vi "element_data_read.vi"(7 "container_name":string, 8 "error in (no error)":errorcluster, 10 "data_type":variant, 11 "Refnum in":T1) -> (0 "error out":errorcluster, 1 "Data Name":string, 2 "data_out":variant, 3 "Refnum out":T1)   [LabVIEW 2015, in "ini_work_Library.lvlib"]
doc: "Created by Artem Shevelev\nshevelev.pro\nartem@shevelev.pro\nLabVIEW Portal: https://labviewportal.org/memberlist.php?mode=viewprofile&u=2340"
uses:
  ini_work_Library.lvlib
  <vilib>/Utility/config.llb/Config Data RefNum.ctl
  <userlib>/_OpenG.lib/lvdata/lvdata.llb/Type Descriptor Enumeration__ogtk.ctl
  <vilib>/Utility/config.llb/Read Key (I32).vi
  <vilib>/Utility/config.llb/Read Key (Double).vi
  <vilib>/Utility/config.llb/Read Key (Boolean).vi
  <vilib>/Utility/config.llb/Read Key (String).vi
  <vilib>/Utility/config.llb/Read Key (Path).vi
  <vilib>/Utility/config.llb/NI_LVConfig.lvlib
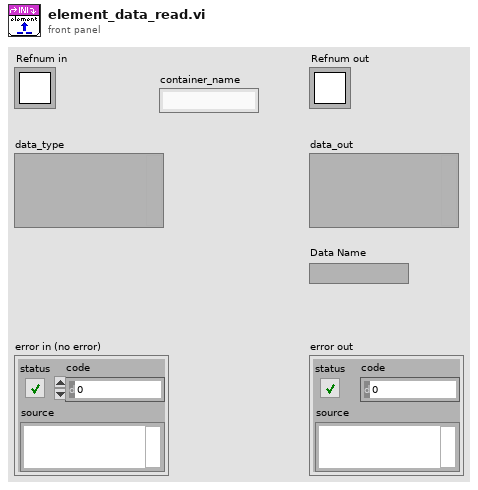
[diagram p1: front panel]
types:
  T1 = typedef "NI_LVConfig.lvlib/Config Data RefNum.ctl" = refnum<k1>
  T2 = typedef "Type Descriptor Enumeration__ogtk.ctl" = enum8{"<Null>", "I8", "I16", "I32", "I64", "U8", "U16", "U32", "U64", "SGL", "DBL", "EXT", "CSG", "CDB", "CXT", "0x0F", "0x10", "0x11", "0x12", "0x13", "0x14", "Enum U8", "Enum U16", "Enum U32", "Enum U64", "SGL PQ", "DBL PQ", "EXT PQ", "CSG PQ", "CDB PQ", "CXT PQ", "0x1F", "0x20", "Boolean", "0x22", "0x23", "0x24", "0x25", "0x26", "0x27", "0x28", "0x29", "0x2A", "0x2B", "0x2C", "0x2D", "0x2E", "0x2F", "String", "0x31", "Path", "Pict", "0x34", "0x35", "0x36", "DAQ", "0x38", "0x39", "0x3A", "0x3B", "0x3C", "0x3D", "0x3E", "0x3F", "Array", "0x41", "0x42", "0x43", "0x44", "0x45", "0x46", "0x47", "0x48", "0x49", "0x4A", "0x4B", "0x4C", "0x4D", "0x4E", "0x4F", "Cluster", "0x51", "0x52", "Variant", "Waveform", "0x55", "0x56", "0x57", "0x58", "0x59", "0x5A", "0x5B", "0x5C", "0x5D", "0x5E", "Fixed Point", "0x60", "0x61", "0x62", "0x63", "0x64", "0x65", "0x66", "0x67", "0x68", "0x69", "0x6A", "0x6B", "0x6C", "0x6D", "0x6E", "0x6F", "Refnum", "0x71", "0x72", "Set Collection", "Map Collection"}
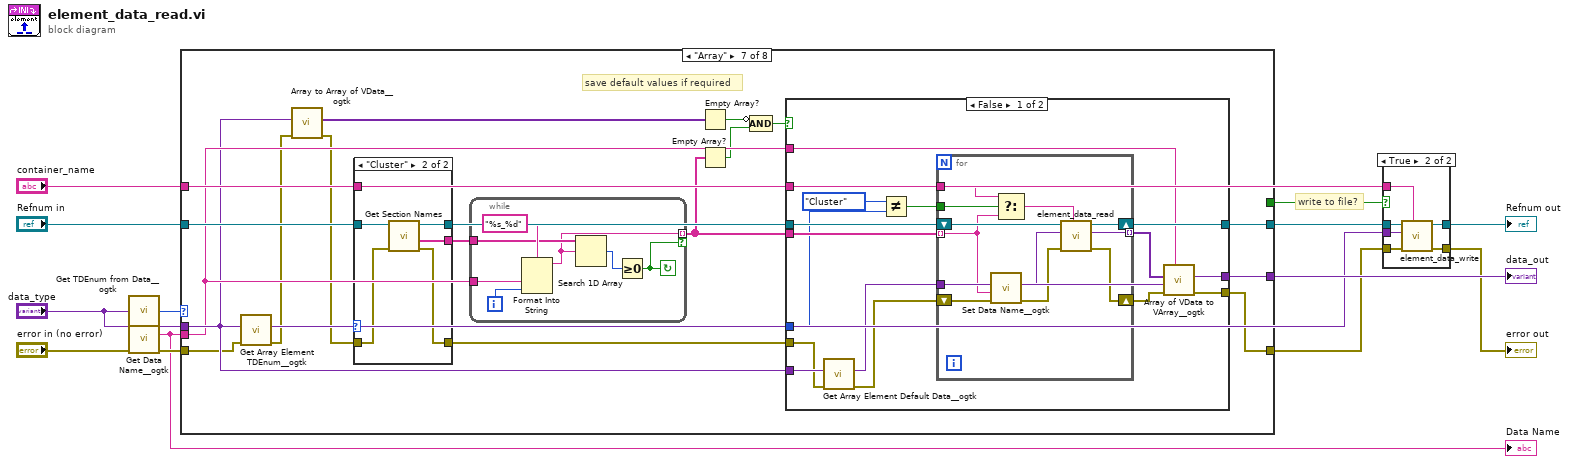
[diagram p0: block diagram]
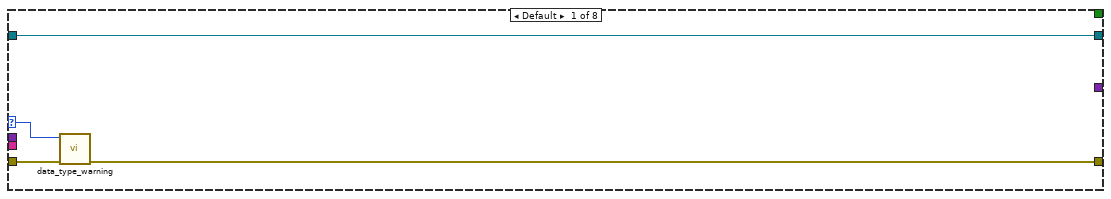
[diagram p3: hidden frame]
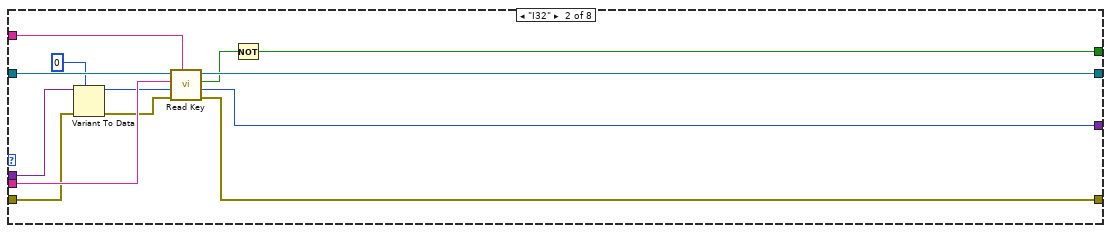
[diagram p4: hidden frame]
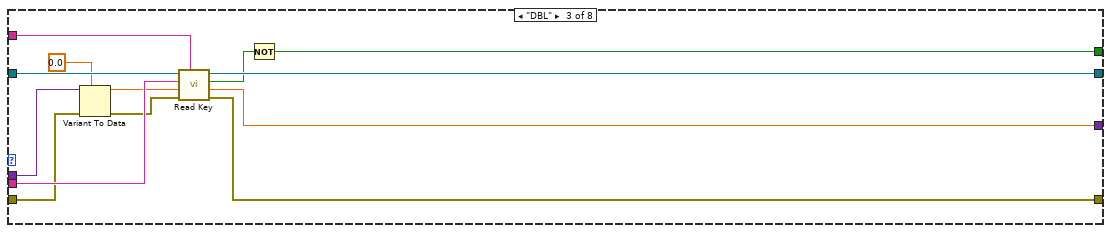
[diagram p5: hidden frame]
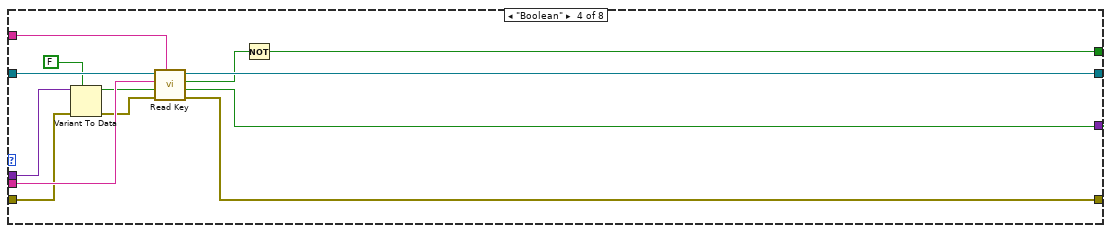
[diagram p6: hidden frame]
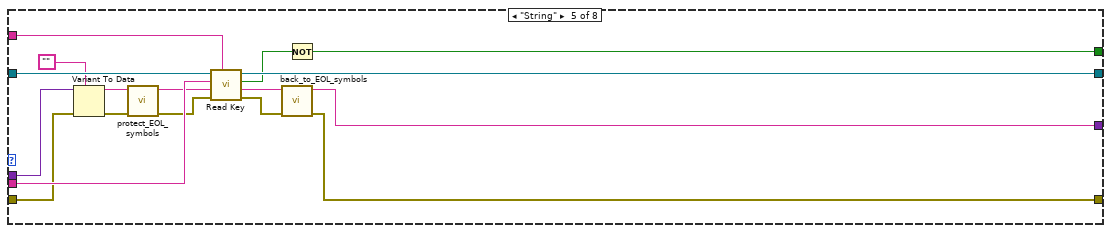
[diagram p7: hidden frame]
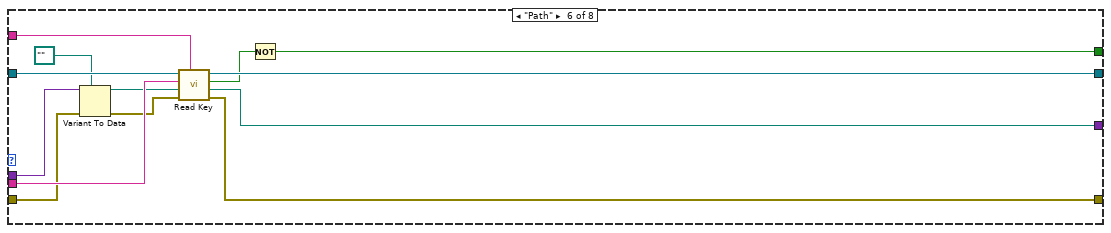
[diagram p8: hidden frame]
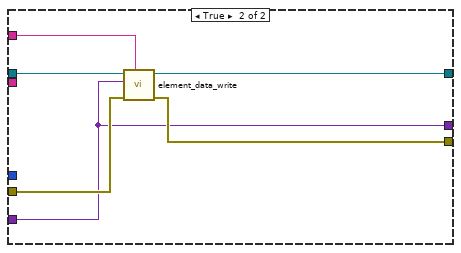
[diagram p9: hidden frame]
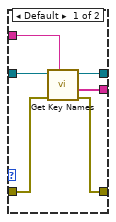
[diagram p10: hidden frame]
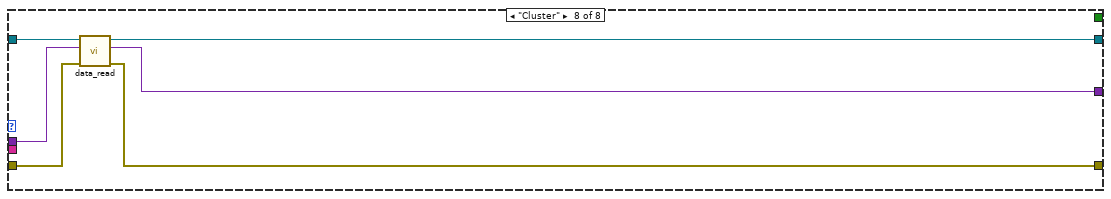
[diagram p11: hidden frame]
diagram:
  # "write to file?"
  n1 = call <userlib>:"Get TDEnum from Data__ogtk.vi"("Data"="data_type") -> ("Type Descriptor Enumeration"=w8:T2)  [unwired: 4 in]
  n2 = call <userlib>:"Get Data Name__ogtk.vi"("error in (no error)"="error in (no error)", "Data"="data_type") -> ("error out"=w13:errorcluster, "Data Name"=w12:string, "Data dup"=w1:variant)  [unwired: 7 in]
  "Data Name" <- w12
  n3 = case shown="\"Array\"" w8 {
    selector: w8 -> [w15 _ _ _ _ _ _ _]
    tunnel: "Refnum in" -> [w17 w31 w44 w57 w74 w87 w106 w164]
    tunnel: w1 -> [_ w21 w39 w55 w72 w86 w92 w162]
    tunnel: w12 -> [_ w30 w42 w56 w73 w85 w94 _]
    tunnel: w13 -> [w18 w27 w38 w52 w70 w82 w90 w161]
    tunnel: "container_name" -> [_ w24 w35 w49 w62 w78 w101 _]
    tunnel: [w17 w25 w36 w50 w61 w79 w99 w163] -> w6
    tunnel: [w16 w23 w34 w48 w60 w80 w102 w159] -> w3
    tunnel: [_ w22 w43 w47 w65 w77 w103 w160] -> w14
    tunnel: [_ w19 w32 w45 w58 w75 _ _] -> w7
    frame Default {
      n4 = call "data_type_warning.vi"("error in (no error)"=w18, "Type Descriptor Enumeration"=w15) -> ("error out"=w16:errorcluster)  [unwired: 9 in]
    }
    frame "I32" {
      n5 = Variant To Data(error in=w27, type=0, Variant=w21) -> (data=w28:i32, error out=w26:errorcluster)
      n6 = call-poly <vilib>:"Read Key.vi"("section"=w24, "error in (no error)"=w26, "default value"=w28, "key"=w30, "refnum"=w31) -> ("error out"=w23:errorcluster, "value"=w22:i32, "found?"=w20:bool, "refnum out"=w25:T1)  [unwired: 3 in]
      n7 = Not(x=w20) -> (.not. x?=w19:bool)
    }
    frame "DBL" {
      n8 = Variant To Data(error in=w38, type=0.0, Variant=w39) -> (data=w40:dbl, error out=w37:errorcluster)
      n9 = call-poly <vilib>:"Read Key.vi"("section"=w35, "error in (no error)"=w37, "default value"=w40, "key"=w42, "refnum"=w44) -> ("error out"=w34:errorcluster, "value"=w43:dbl, "found?"=w33:bool, "refnum out"=w36:T1)  [unwired: 3 in]
      n10 = Not(x=w33) -> (.not. x?=w32:bool)
    }
    frame "Boolean" {
      n11 = Variant To Data(error in=w52, type=FALSE, Variant=w55) -> (data=w53:bool, error out=w51:errorcluster)
      n12 = call-poly <vilib>:"Read Key.vi"("section"=w49, "error in (no error)"=w51, "default value"=w53, "key"=w56, "refnum"=w57) -> ("error out"=w48:errorcluster, "value"=w47:bool, "found?"=w46:bool, "refnum out"=w50:T1)  [unwired: 3 in]
      n13 = Not(x=w46) -> (.not. x?=w45:bool)
    }
    frame "String" {
      n14 = Variant To Data(error in=w70, type="", Variant=w72) -> (data=w67:string, error out=w69:errorcluster)
      n15 = call "protect_EOL_symbols.vi"("error in (no error)"=w69, "String"=w67) -> ("error out"=w68:errorcluster, "result string"=w66:string)  [unwired: 8 in]
      n16 = call-poly <vilib>:"Read Key.vi"("section"=w62, "error in (no error)"=w68, "default value"=w66, "key"=w73, "refnum"=w74) -> ("error out"=w63:errorcluster, "value"=w64:string, "found?"=w59:bool, "refnum out"=w61:T1)  [unwired: 3 in]
      n17 = call "back_to_EOL_symbols.vi"("error in (no error)"=w63, "value"=w64) -> ("error out"=w60:errorcluster, "result string"=w65:string)  [unwired: 8 in]
      n18 = Not(x=w59) -> (.not. x?=w58:bool)
    }
    frame "Path" {
      n19 = Variant To Data(error in=w82, type=path "" ("default value"), Variant=w86) -> (data=w83:path, error out=w81:errorcluster)
      n20 = call-poly <vilib>:"Read Key.vi"("section"=w78, "error in (no error)"=w81, "default value"=w83, "key"=w85, "refnum"=w87) -> ("error out"=w80:errorcluster, "value"=w77:path, "found?"=w76:bool, "refnum out"=w79:T1)  [unwired: 3 in]
      n21 = Not(x=w76) -> (.not. x?=w75:bool)
    }
    frame "Array" {
      # "save default values if required"
      n22 = call <userlib>:"Get Array Element TDEnum__ogtk.vi"("error in (no error)"=w90, "Array"=w92) -> ("error out"=w89:errorcluster, "Element Type"=w93:T2)  [unwired: 8 in]
      n23 = call <userlib>:"Array to Array of VData__ogtk.vi"("error in (no error)"=w89, "MultiD Array"=w92) -> ("error out"=w88:errorcluster, "1D Array of Variants"=w95:variant[])  [unwired: 8 in]
      n24 = case shown="\"Cluster\"" w93 {
        tunnel: w106 -> [w153 w158]
        tunnel: w88 -> [w151 w157]
        tunnel: w101 -> [w152 _]
        tunnel: [w150 w156] -> w105
        tunnel: [w148 w155] -> w104
        tunnel: [w149 w154] -> w100
        frame Default {
          n25 = call <vilib>:"Get Key Names.vi"("section"=w152, "error in (no error)"=w151, "refnum"=w153) -> ("error out"=w148:errorcluster, "key names"=w149:string[], "refnum out"=w150:T1)  [unwired: 5 in, 1 out]
        }
        frame "Cluster" {
          n26 = call <vilib>:"Get Section Names.vi"("error in (no error)"=w157, "refnum"=w158) -> ("error out"=w155:errorcluster, "section names"=w154:string[], "refnum out"=w156:T1)  [unwired: 7 in]
        }
      }
      n27 = while {
        tunnel: w100 -> [w144]
        tunnel: w94 -> [w145]
        tunnel: [w143] -> w98 mode=indexing if=w141
        i -> [w146]
        stop <- w141 continue-if-true
        n28 = Format Into String(format string="%s_%d", w145, w146) -> (resulting string=w143:string)  [unwired: 2 in, 1 out]
        n29 = Search 1D Array(1D array=w144, element=w143) -> (index of element=w142:i32)  [unwired: 1 in]
        n30 = Greater Or Equal To 0?(x=w142) -> (x >= 0?=w141:bool)
      }
      n31 = Empty Array?(array=w95) -> (empty?=w97:bool)
      n32 = Empty Array?(array=w98) -> (empty?=w91:bool)
      n33 = Compound Arithmetic op=AND(invert w97, w91) -> (w96:bool)
      n34 = case shown="False" w96 {
        tunnel: w105 -> [w122 w140]
        tunnel: w104 -> [w111 w137]
        tunnel: w93 -> [w108 _]
        tunnel: [w114 w135] -> w103
        tunnel: [w115 w136] -> w102
        tunnel: w101 -> [w121 w138]
        tunnel: [w120 w139] -> w99
        tunnel: w98 -> [w119 _]
        tunnel: w92 -> [w113 w135]
        tunnel: w94 -> [w116 _]
        frame False {
          n35 = call <userlib>:"Get Array Element Default Data__ogtk.vi"("error in (no error)"=w111, "Array"=w113) -> ("error out"=w110:errorcluster, "Array Element Default Data"=w112:variant)  [unwired: 8 in]
          n36 = Not Equal?(x=Type_Descriptor_Enumeration__ogtk."Cluster" ("Element Type"), y=w108) -> (x != y?=w107:bool)
          n37 = for {
            shift-right: [w133] -> w120
            shift-left: w122 -> [w134]
            shift-right: [w129] -> w117
            shift-left: w110 -> [w131]
            tunnel: w119 -> [w125] mode=indexing
            tunnel: w112 -> [w132]
            tunnel: [w130] -> w118 mode=indexing
            tunnel: w121 -> [w124]
            tunnel: w107 -> [w126]
            n38 = call <userlib>:"Set Data Name__ogtk.vi"("error in (no error)"=w131, "Data Name"=w125, "Data"=w132) -> ("error out"=w128:errorcluster, "Renamed Data"=w127:variant)  [unwired: 7 in]
            n39 = Select(t=w124, s=w126, f=w125) -> (s? t:f=w123:string)
            n40 = call "element_data_read.vi"("container_name"=w123, "error in (no error)"=w128, "data_type"=w127, "Refnum in"=w134) -> ("error out"=w129:errorcluster, "data_out"=w130:variant, "Refnum out"=w133:T1)  [unwired: 4 in, 1 out]
          }
          n41 = call <userlib>:"Array of VData to VArray__ogtk.vi"("Array Name"=w116, "error in (no error)"=w117, "Element Type (when empty)"=w112, "1D Array of VData"=w118) -> ("error out"=w115:errorcluster, "VArray"=w114:variant)  [unwired: 6 in]
        }
        frame True {
          n42 = call "element_data_write.vi"("container_name"=w138, "error in (no error)"=w137, "Variant"=w135, "Refnum in"=w140) -> ("error out"=w136:errorcluster, "Refnum out"=w139:T1)  [unwired: 6 in]
        }
      }
    }
    frame "Cluster" {
      n43 = call "data_read.vi"("error in (no error)"=w161, "dataContainer"=w162, "ini_file_refnum"=w164) -> ("error out"=w159:errorcluster, "dataValue"=w160:variant, "ini_file_refnum_out"=w163:T1)  [unwired: 6 in]
    }
  }
  "data_out" <- w14
  n44 = case shown="True" w7 {
    tunnel: w6 -> [w166 w172]
    tunnel: [w166 w171] -> w5
    tunnel: "container_name" -> [_ w170]
    tunnel: w3 -> [w165 w169]
    tunnel: [w165 w168] -> w2
    tunnel: w1 -> [_ w167]
    frame False {
    }
    frame True {
      n45 = call "element_data_write.vi"("container_name"=w170, "error in (no error)"=w169, "Variant"=w167, "Refnum in"=w172) -> ("error out"=w168:errorcluster, "Refnum out"=w171:T1)  [unwired: 6 in]
    }
  }
  "error out" <- w2
  "Refnum out" <- w5
